vi "GetType.vi"(8 "error in (no error)":errorcluster, 11 "Send Software Advanced Trigger [AT] Msg":refnum<class "Send Software Advanced Trigger [AT] Msg.lvclass">) -> (0 "error out":errorcluster, 2 "Data Sample":variant, 3 "Send Software Advanced Trigger [AT] Msg":refnum<class "Send Software Advanced Trigger [AT] Msg.lvclass">)   [LabVIEW 2015, in "CS++Fgen.lvlib" / "Send Software Advanced Trigger [AT] Msg.lvclass"]
doc: "This VI delivers a sample of the data type format the message expects."
uses:
  Send Software Advanced Trigger [AT] Msg.lvclass
  Send Software Advanced Trigger [AT] Msg.lvclass/Send Software Advanced Trigger [AT] Msg.ctl
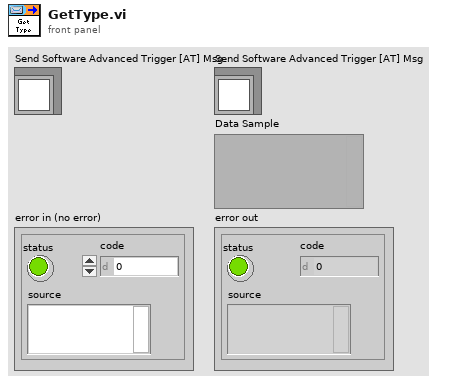
[diagram p1: front panel]
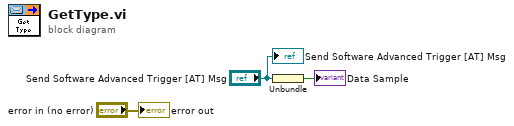
[diagram p0: block diagram]
diagram:
  n1 = Unbundle("Send Software Advanced Trigger [AT] Msg") -> (→"Data Sample":bool)
  "error out" <- "error in (no error)"
  "Send Software Advanced Trigger [AT] Msg" <- "Send Software Advanced Trigger [AT] Msg"
